vi "Sett_UP_Convert.vi"(8 "error in (no error)":errorcluster, 9 "Divider(1)":dbl=1.0, 11 "ISO 15693 DOWN in":refnum<class "ISO 15693 DOWN.lvclass">) -> (0 "error out":errorcluster, 2 "Waveform":waveform(dbl), 3 "ISO 15693 DOWN out":refnum<class "ISO 15693 DOWN.lvclass">)   [LabVIEW 2019, in "ISO 15693 DOWN.lvclass"]
uses:
  ISO 15693 DOWN.lvclass
  ISO 15693 DOWN.lvclass/ISO 15693 DOWN.ctl
  <vilib>/addons/Modulation/Analog/support/mod_Set Error Source.vi
  <vilib>/addons/Modulation/Digital/Support/Common/Validators/mod_Generate Filter Coefficients Validate.vi
  <vilib>/addons/Modulation/Digital/General/subVIs/mod_Generate Filter Coefficients.vi
  <vilib>/addons/Modulation/Digital/General/MT Generate ASK system parameters (M).vi
  <vilib>/addons/Modulation/niDMT.lvlib
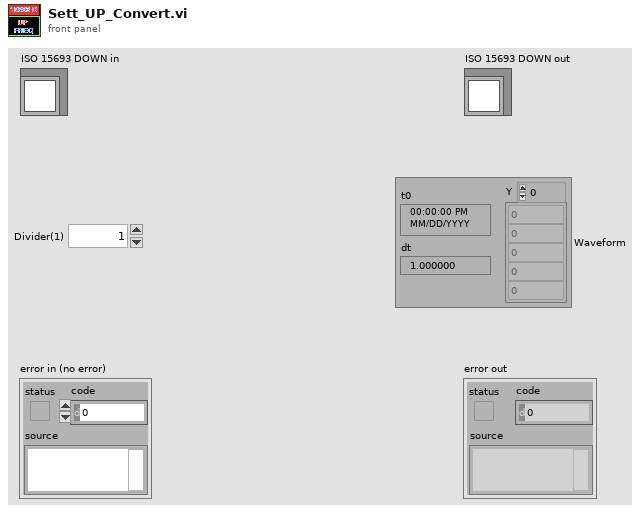
[diagram p1: front panel]
types:
  T1 = enum16{"none", "Raised Cosine", "Root Raised Cos", "Gaussian"}
  T2 = enum16{"FSK", "PSK", "QAM", "MSK", "PAM", "ASK", "CPM"}
  T3 = cluster{"samples per symbol (16)":i32, "symbol map":cdb[]}
  T4 = typedef "niAMT.lvlib/Complex Data Waveform.ctl" = cluster{"t0":dbl, "dt":dbl, "Y":cdb[]}
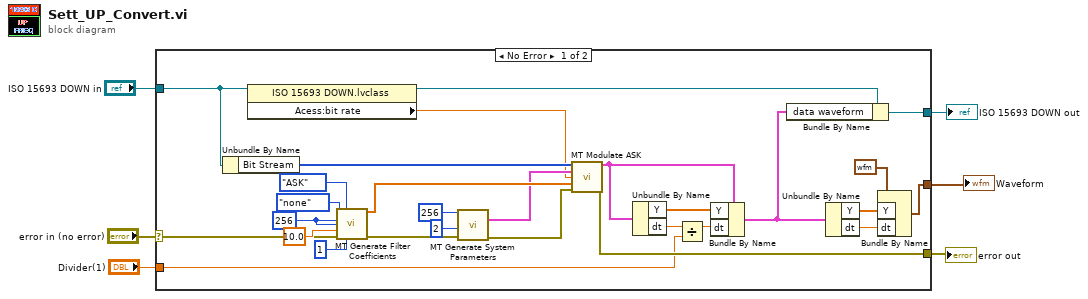
[diagram p0: block diagram]
diagram:
  n1 = case shown="No Error" "error in (no error)" {
    selector: "error in (no error)" -> [w9 w36]
    tunnel: "ISO 15693 DOWN in" -> [w13 w35]
    tunnel: [w12 w35] -> w5
    tunnel: [w11 _] -> w1
    tunnel: [w10 w36] -> w4
    tunnel: "Divider(1)" -> [w8 _]
    frame No Error {
      w27 = 256 ("pulse shaping samples per symbol (16)")
      n2 = Unbundle By Name(w13) -> ("Bit Stream"=w20:u8[])
      n3 = property class="ISO 15693 DOWN.lvclass"(reference=w13) -> (reference out=w14:refnum<class "ISO 15693 DOWN.lvclass">, "Acess:bit rate"=w15:dbl)  [unwired: 1 in, 1 out]
      n4 = call <vilib>:"MT Generate Filter Coefficients.vi"("pulse shaping filter (none)"=T1."none", "modulation type"=T2."ASK", "pulse shaping samples per symbol (16)"=w27, "matched samples per symbol (16)"=w27, "filter parameter"=10.0, "error in (no error)"=w9, "filter length (symbols)"=1) -> ("pulse shaping filter coefficients"=w29:dbl[], "error out"=w24:errorcluster)  [unwired: 7 out]
      n5 = call-poly <vilib>:"MT Generate System Parameters.vi"("samples per symbol (16)"=256, "M-ASK (2)"=2, "error in (no error)"=w24) -> ("ASK system parameters"=w21:T3, "error out"=w22:errorcluster)  [unwired: 11 out]
      n6 = call <vilib>:"MT Modulate ASK.vi"("input bit stream"=w20, "ASK system parameters"=w21, "symbol rate (Hz)"=w15, "pulse shaping filter coefficients"=w29, "error in (no error)"=w22) -> ("output complex waveform"=w19:T4, "error out"=w10:errorcluster)  [unwired: 8 in, 1 out]
      n7 = Unbundle By Name(w19) -> ("Y"=w32:cdb[], "dt"=w34:dbl)
      n8 = Divide(x=w34, y=w8) -> (x/y=w33:dbl)
      n9 = Bundle By Name(cluster=w19, "Y"=w32, "dt"=w33) -> (w16:T4)
      n10 = Bundle By Name(cluster=w14, "data waveform"=w16) -> (w12:refnum<class "ISO 15693 DOWN.lvclass">)
      n11 = Unbundle By Name(w16) -> ("Y"=w18:cdb[], "dt"=w17:dbl)
      n12 = Bundle By Name(cluster=waveform(dbl) {"t0"=timestamp(0 s since 1904-01-01), "dt"=0.0, "Y"=array[8576 elements]} ("Waveform"), "Y"=w18, "dt"=w17) -> (w11:waveform(dbl))
    }
    frame Error {
    }
  }
  "error out" <- w4
  "ISO 15693 DOWN out" <- w5
  "Waveform" <- w1
